vi "PH_Beckhoff_PPMA-Rods.set Safe State.vi"(0 "i ref in":refnum<vi>, 5 "error in":errorcluster) -> (14 "i ref out":refnum<vi>, 19 "error out":errorcluster)   [LabVIEW 2014, in "PH_Beckhoff_PPMA-Rods.lvlib"]
doc: "This VI calls several simple event calls to set the hardware to a safe (default) state. It is supposed to be used in con- and destructor."
uses:
  PH_Beckhoff_PPMA-Rods.lvlib
  CSCore/CSSystem/CSSystemLib/CSSystemLib.lvlib
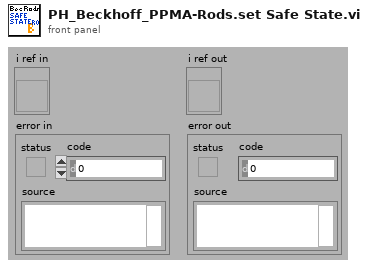
[diagram p1: front panel]
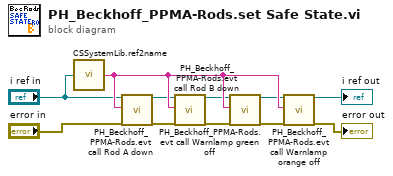
[diagram p0: block diagram]
diagram:
  n1 = call "CSSystemLib.ref2name.vi"("obj refnum"="i ref in") -> ("name"=w10:string)
  n2 = call "PH_Beckhoff_PPMA-Rods.evt call Rod A down.vi"("i ref in"="i ref in", "Instance name"=w10, "error in"="error in") -> ("i ref out"=w3:refnum<vi>, "error out"=w5:errorcluster)  [unwired: 15 in]
  n3 = call "PH_Beckhoff_PPMA-Rods.evt call Rod B down.vi"("i ref in"=w3, "Instance name"=w10, "error in"=w5) -> ("i ref out"=w2:refnum<vi>, "error out"=w6:errorcluster)  [unwired: 15 in]
  n4 = call "PH_Beckhoff_PPMA-Rods.evt call Warnlamp green off.vi"("i ref in"=w2, "Instance name"=w10, "error in"=w6) -> ("i ref out"=w1:refnum<vi>, "error out"=w4:errorcluster)  [unwired: 15 in]
  n5 = call "PH_Beckhoff_PPMA-Rods.evt call Warnlamp orange off.vi"("i ref in"=w1, "Instance name"=w10, "error in"=w4) -> ("i ref out"=→"i ref out":refnum<vi>, "error out"=→"error out":errorcluster)  [unwired: 15 in]
